vi "getPayloadRequirement.vi"(11 "CONNECT in":refnum<class "CONNECT.lvclass">) -> (2 "Requirement":T1, 3 "CONNECT out":refnum<class "CONNECT.lvclass">)   [LabVIEW 2013, in "MQTT_Control_Packets.lvlib" / "CONNECT.lvclass"]
uses:
  CONNECT.lvclass
  ControlPacket/Requirement -- enum.ctl
  ControlPacket/ControlPacket.lvclass
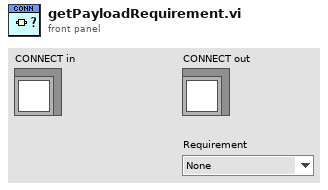
[diagram p1: front panel]
types:
  T1 = typedef "MQTT_Control_Packets.lvlib/ControlPacket.lvclass/Requirement -- enum.ctl" = enum16{"None", "Optional", "Required"}
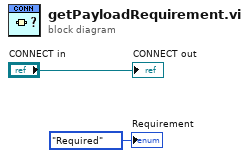
[diagram p0: block diagram]
diagram:
  "CONNECT out" <- "CONNECT in"
  "Requirement" <- Requirement_--_enum."Required" ("Requirement")
